vi "logistic_fn.vi"(11 "Input":dbl) -> (3 "Output":dbl, 7 "Waveform Chart":cluster{dbl}(graph))   [LabVIEW 2014]
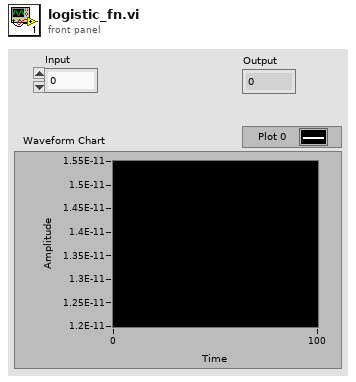
[diagram p1: front panel]
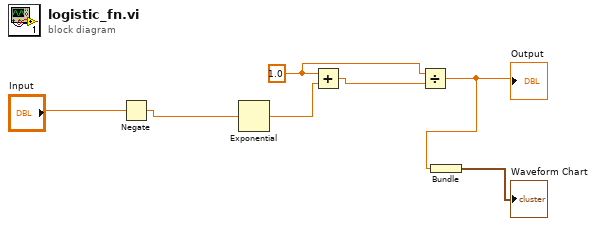
[diagram p0: block diagram]
diagram:
  w5 = 1.0 ("x")
  n1 = Negate(x="Input") -> (-x=w7:dbl)
  n2 = Exponential(1:w7) -> (0:w6:dbl)
  n3 = Add(x=w5, y=w6) -> (x+y=w4:dbl)
  n4 = Divide(x=w5, y=w4) -> (x/y=w2:dbl)
  "Output" <- w2
  n5 = Bundle(w2) -> (→"Waveform Chart":cluster{dbl})  [unwired: 1 in]
